vi "Read Test Case.vi"(11 "Test Case Result In":refnum<class "Test Case Result.lvclass">) -> (2 "Test Case":string, 3 "Test Case Result Out":refnum<class "Test Case Result.lvclass">)   [LabVIEW 2020, in "Test Case Result.lvclass"]
uses:
  Test Case Result.lvclass
  Test Case Result.lvclass/Test Case Result.ctl
  Method Result/Method Result.lvclass/Method Result.ctl
  Method Result/Method Result.lvclass
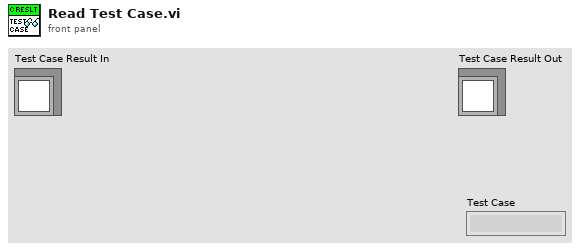
[diagram p1: front panel]
types:
  T1 = map{string, refnum<class "Method Result.lvclass">}
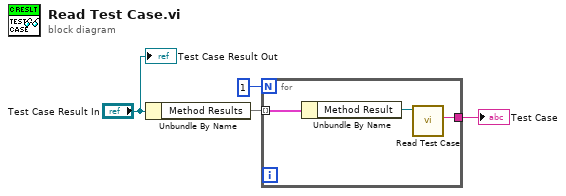
[diagram p0: block diagram]
diagram:
  n1 = Unbundle By Name("Test Case Result In") -> ("Method Results"=w3:T1)
  n2 = for {
    N: 1 -> [_]
    tunnel: w3 -> [w6] mode=indexing
    tunnel: [w7] -> w1
    n3 = Unbundle By Name(w6) -> ("Method Result"=w5:refnum<class "Method Result.lvclass">)
    n4 = call "Read Test Case.vi"("Method Result In"=w5) -> ("Test Case"=w7:string)  [unwired: 9 in, 1 out]
  }
  "Test Case" <- w1
  "Test Case Result Out" <- "Test Case Result In"
